vi "Run Action.vi"(7 "Logger":refnum<class "Logger.lvclass">, 8 "error in (no error)":errorcluster, 10 "Package":refnum<class "PackageAbstract.lvclass">, 11 "InitAction in":refnum<class "InitAction.lvclass">) -> (0 "error out":errorcluster, 2 "Problems":string[](array[string]), 3 "InitAction out":refnum<class "InitAction.lvclass">)   [LabVIEW 2020, in "GPackTools.lvlib" / "InitAction.lvclass"]
uses:
  InitAction.lvclass
  GPack/PackageAbstract/PackageAbstract.lvclass
  GPack/Logger/Logger.lvclass
  InitAction.lvclass/InitAction.ctl
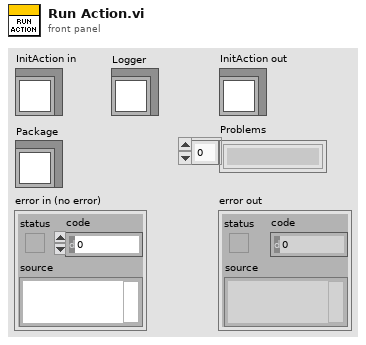
[diagram p1: front panel]
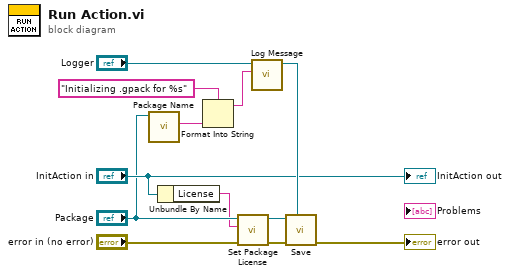
[diagram p0: block diagram]
diagram:
  n1 = call-dynamic "Package Name.vi"("PackageInfo in"="Package") -> ("Package Name"=w8:string)  [unwired: 9 in, 1 out]
  n2 = Unbundle By Name("InitAction in") -> ("License"=w1:string)
  n3 = Format Into String(format string="Initializing .gpack for %s", w8) -> (resulting string=w6:string)  [unwired: 2 in, 1 out]
  n4 = call-dynamic "Set Package License.vi"("error in (no error)"="error in (no error)", "License"=w1, "PackageInfo in"="Package") -> ("error out"=w4:errorcluster, "PackageInfo out"=w3:refnum<class "PackageAbstract.lvclass">)  [unwired: 7 in]
  n5 = call "Log Message.vi"("Message"=w6, "Logger in"="Logger") -> ("Logger out"=w7:refnum<class "Logger.lvclass">)  [unwired: 8 in, 1 out]
  n6 = call "Save.vi"("Logger"=w7, "error in (no error)"=w4, "PackageAbstract in"=w3) -> ("error out"=→"error out":errorcluster)  [unwired: 7 in, 1 out]
  "InitAction out" <- "InitAction in"
